vi "VI_FP prepare for run.vi"(8 "error in (no error)":errorcluster, 11 "VI in":refnum<vi>) -> (0 "error out":errorcluster, 3 "VI out":refnum<vi>)   [LabVIEW 2015]
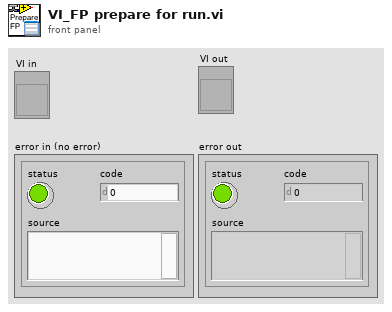
[diagram p1: front panel]
types:
  T1 = enum32{"Invalid", "Standard", "Closed", "Hidden", "Minimized", "Maximized"}
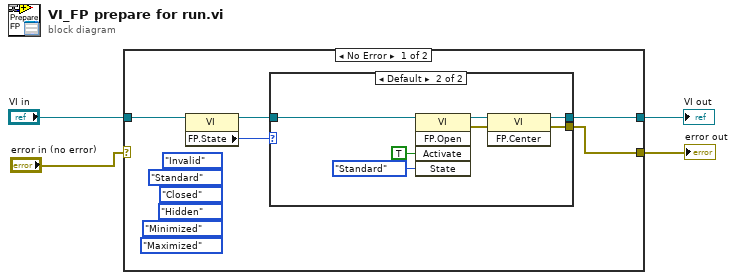
[diagram p0: block diagram]
diagram:
  n1 = case shown="No Error" "error in (no error)" {
    selector: "error in (no error)" -> [_ w18]
    tunnel: [w9 w19] -> w4
    tunnel: "VI in" -> [w7 w19]
    tunnel: [w8 w18] -> w1
    frame No Error {
      (unwired) T1."Maximized" ("Front Panel Window:State")
      (unwired) T1."Minimized" ("Front Panel Window:State")
      (unwired) T1."Hidden" ("Front Panel Window:State")
      (unwired) T1."Closed" ("Front Panel Window:State")
      (unwired) T1."Standard" ("Front Panel Window:State")
      (unwired) T1."Invalid" ("Front Panel Window:State")
      n2 = property class="VI"(reference=w7) -> (reference out=w6:refnum<vi>, "FP.State"=w5:T1)  [unwired: 1 in, 1 out]
      n3 = case shown="Default" w5 {
        tunnel: [w10 w14] -> w9
        tunnel: [_ w12] -> w8
        tunnel: w6 -> [w10 w11]
        frame "Standard" {
        }
        frame Default {
          n4 = invoke class="VI" method="FP.Open"(reference=w11, "Activate"=TRUE ("Activate?"), "State"=T1."Standard") -> (reference out=w15:refnum<vi>, error out=w13:errorcluster)  [unwired: 2 in, 3 out]
          n5 = invoke class="VI" method="FP.Center"(reference=w15, error in=w13) -> (reference out=w14:refnum<vi>, error out=w12:errorcluster)  [unwired: 1 in, 1 out]
        }
      }
    }
    frame Error {
    }
  }
  "VI out" <- w4
  "error out" <- w1
